vi "Get_Ai_2D_array.vi"(0 "reference in":refnum<class "FPGA_Interface.lvclass">, 11 "error in (no error)":errorcluster) -> (4 "reference out":refnum<class "FPGA_Interface.lvclass">, 6 "AIs":dbl[][](array[numeric]), 8 "data valid":bool, 15 "error out":errorcluster)   [LabVIEW 2019, in "FPGA_Interface.lvclass"]
uses:
  FPGA_Interface.lvclass
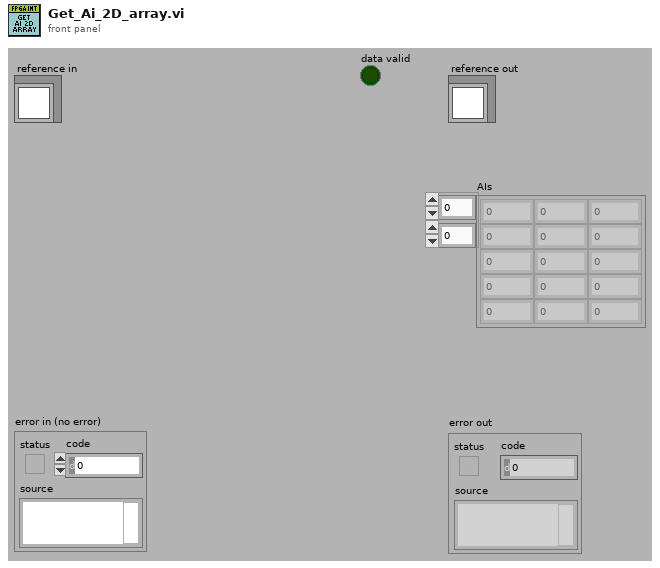
[diagram p1: front panel]
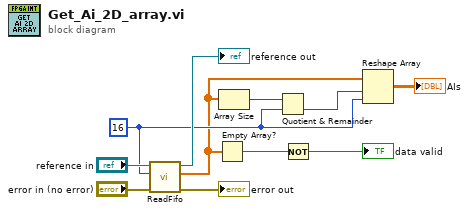
[diagram p0: block diagram]
diagram:
  w4 = 16 ("N")
  n1 = call-dynamic "ReadFifo.vi"("error in (no error)"="error in (no error)", "N"=w4, "FPGA_Interface in"="reference in") -> ("error out"=→"error out":errorcluster, "Data"=w3:dbl[], "FPGA_Interface out"=→"reference out":refnum<class "FPGA_Interface.lvclass">)  [unwired: 6 in]
  n2 = Empty Array?(array=w3) -> (empty?=w2:bool)
  n3 = Array Size(array=w3) -> (size(s)=w6:i32)
  n4 = Quotient & Remainder(x=w6, y=w4) -> (floor(x/y)=w5:i32)  [unwired: 1 out]
  n5 = Not(x=w2) -> (.not. x?=→"data valid":bool)
  n6 = Reshape Array(w3, w5, w4) -> (→"AIs":dbl[][])
